vi "Gyro Example.vi"() -> ()   [LabVIEW 2011]
doc: "Gyro Example\n\nThis VI shows the user how to open a channel to a Gyro, get an angle from a gyro, and reinitialize the gyro."
uses:
  <vilib>/Rock Robotics/SystemInterfaces/AI/FPGA_AIGyroChannel.ctl
  <vilib>/Rock Robotics/WPI/Joystick/WPI_JoystickDeviceEnum.ctl
  <vilib>/Rock Robotics/WPI/RobotDrive/WPI_RobotDriveOpen4MotorWithCANJaguar.vi
  <vilib>/Rock Robotics/WPI/RobotDrive/WPI_RobotDriveArcadeDrive_Standard(NoSaturation).vi
panel:
  out "X-Axis Out":dbl(slide) scale=-1.0..1.0
  in  "Analog Channel":T1=enum."AI 2"
  in  "Gain (VoltsPerDegree/Second)":dbl=0.0068
  in  "stop":bool
  out "Angle":dbl(knob) scale=0.0..360.0
  in  "Reset Zero Position":bool
  # "This will display the current gyro angle."
  # "Wiring Diagram for Analog Breakout connected to an NI 9201"
  # "Set these inputs before running."
  # "This can be set while running."
  # "jumper to read battery or AI8"
  # "GND"
  # "SIG"
  # "5V"
  # "AI8\nAI7\nAI6\nAI5\nAI4\nAI3\nAI2\nAI1"
  # "Generic Gyro"
  # "+"
  # "12V from battery"
  # "-"
  # "default 0.0125\n0.00665 - close (within ~3 deg of 90 rot)\n0.00680 - (within ~19 of 360 rot)"
  # "\"power good\" LED"
  # "Specific Gyro Wiring:\nFor Analog Devices ADXRS401EB, ADXRS150EB and ADXRS300EB, wire RATEOUT to AI1 SIG (white PWM wire), wire AGND to AI1 GND (black PWM wire), and wire AVCC to AI1 5V (PWM red wire).  Also wire from AVCC to PDD.\n\nMost SparkFun Gyros wire according to the generic diagram"
  # "RATE"
  # "5V"
  # "GND"
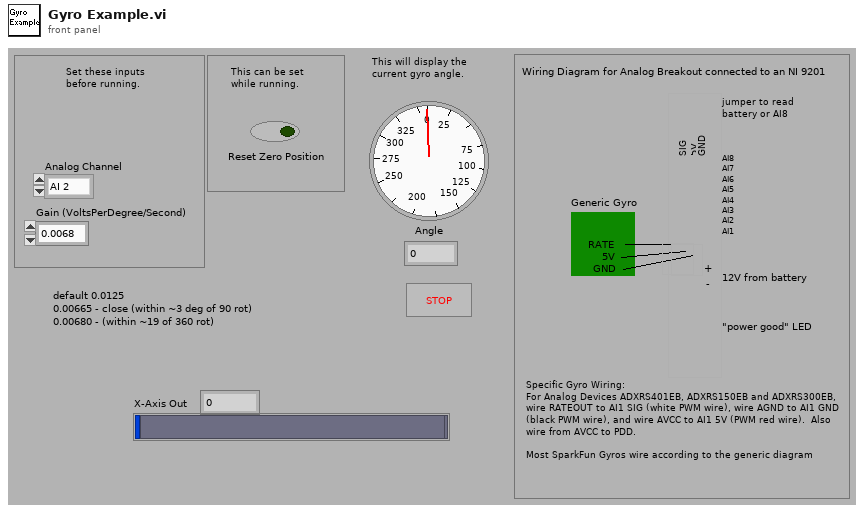
[diagram p1: front panel]
types:
  T1 = typedef "FPGA_AIGyroChannel.ctl" = enum8{"AI 1", "AI 2", "Invalid"}
  T2 = typedef "WPI_JoystickDeviceEnum.ctl" = enum16{"USB 1", "USB 2", "USB 3", "USB 4", "Kinect 1", "Kinect 2"}
  T3 = typedef "WPI_RobotDriveDevRef.ctl" = cluster{"DevStatus":errorcluster, "Motors[]":T4[], "Square Inputs":bool, "Max Output":dbl, "Isochronous":bool}
  T4 = typedef "WPI_MotorControlDeviceRef.ctl" = cluster{"DeviceStatus":errorcluster, "Type":enum16{"PWM", "CAN"}, "PWM":cluster{"Digital Module":T5, "PWM Channel":T6, "DeadBand":T7}, "CAN":cluster{"Device Number":u8, "Control Mode":T8, "Semaphore":T9, "Max Vout":dbl}, "Invert":bool, "TransformRef":T10, "InvTransformRef":T10}
  T5 = typedef "FPGA_TypedefDigitalModule.ctl" = enum16{"Digital Module 1", "Digital Module 2"}
  T6 = typedef "FPGA_DIOPWMChannel.ctl" = enum8{"PWM 1", "PWM 2", "PWM 3", "PWM 4", "PWM 5", "PWM 6", "PWM 7", "PWM 8", "PWM 9", "PWM 10", "Invalid"}
  T7 = typedef "WPI_PWMDeadband.ctl" = cluster{"Name":string, "maxPositivePwm":i32, "minPositivePwm":i32, "centerPwm":i32, "maxNegativePwm":i32, "minNegativePwm":i32, "angularRange":u16}
  T8 = typedef "WPI_CANJaguar_ControlMode.ctl" = enum8{"Percent VBus", "Current", "Speed", "Position", "Voltage"}
  T9 = typedef "Semaphore RefNum" = refnum<k1>
  T10 = typedef "WPI_PWMTransform_ConPane.ctl" = refnum<vi>
  T11 = typedef "WPI_GyroDevRef.ctl" = cluster{"DevStatus":errorcluster, "Analog Module":T12, "Analog Channel":T13, "Offset":dbl, "Gain (VoltsPerDegree/Second)":dbl}
  T12 = typedef "FPGA_TypedefAnalogModule.ctl" = enum16{"Analog Module 1", "Analog Module 2"}
  T13 = typedef "FPGA_AIChannel.ctl" = enum8{"AI 1", "AI 2", "AI 3", "AI 4", "AI 5", "AI 6", "AI 7", "AI 8", "Invalid"}
  T14 = typedef "WPI_JoystickDevRef.ctl" = cluster{"Device":T2}
  T15 = cluster{"axis 1 (x)":dbl, "axis 2 (y)":dbl, "axis 3 (throttle)":dbl, "axis 4":dbl, "axis 5":dbl, "axis 6":dbl}
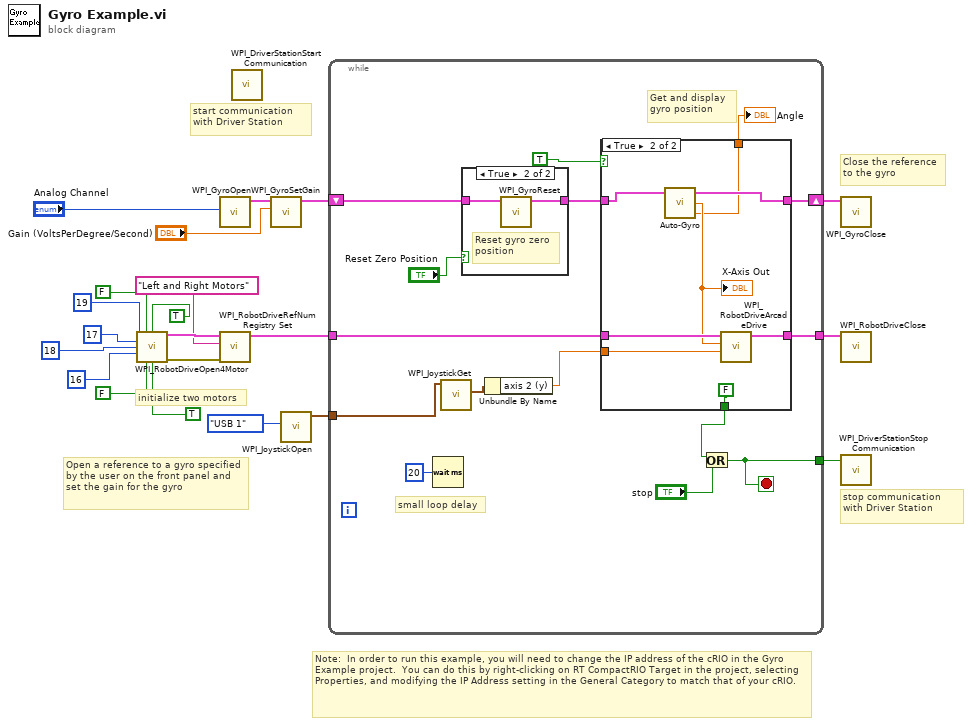
[diagram p0: block diagram]
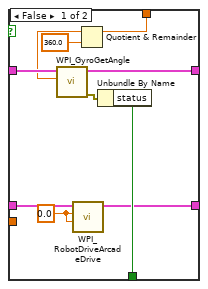
[diagram p2: hidden frame]
diagram:
  # "initialize two motors"
  # "stop communication with Driver Station"
  # "start communication with Driver Station"
  # "Note:  In order to run this example, you will need to change the IP address of the cRIO in the Gyro Example project.  You can do this by right-clicking on RT CompactRIO Target in the project, selecting Properties, and modifying the IP Address setting in the General Category to match that of your cRIO."
  # "Close the reference\nto the gyro"
  # "Open a reference to a gyro specified by the user on the front panel and set the gain for the gyro"
  n1 = call-poly <vilib>:"WPI_RobotDriveOpen4Motor.vi"("Rear Left Motor"=u8 19, "Rear Left Motor Inverted"=FALSE, "Rear Right Motor Inverted"=TRUE ("Rear Left Motor Inverted"), "Rear Right Motor"=u8 17, "Front Left Motor"=u8 18, "Front Right Motor"=u8 16, "Front Left Motor Inverted"=FALSE, "Front Right Motor Inverted"=TRUE) -> ("RobotDriveDevRef"=w15:T3, "error out"=w13:errorcluster)  [unwired: 6 in]
  n2 = call <vilib>:"WPI_GyroOpen.vi"("Analog Channel"="Analog Channel") -> ("GyroDevRef"=w19:T11)  [unwired: 5 in, 5 out]
  n3 = call <vilib>:"WPI_RobotDriveRefNum Registry Set.vi"("error in (no error)"=w13, "refnum name"="Left and Right Motors", "RobotDriveDevRef"=w15) -> ("RobotDriveDevRef"=w4:T3)  [unwired: 8 out]
  n4 = call <vilib>:"WPI_DriverStationStart Communication.vi"() -> ()  [unwired: 1 in, 11 out]
  n5 = call <vilib>:"WPI_GyroSetGain.vi"("Gain (VoltsPerDegree/Second)"="Gain (VoltsPerDegree/Second)", "GyroDevRef"=w19) -> ("GyroDevRef"=w18:T11)  [unwired: 1 in, 8 out]
  n6 = call <vilib>:"WPI_JoystickOpen.vi"("JoystickDevice"=WPI_JoystickDeviceEnum."USB 1") -> ("JoystickDevRef"=w1:T14)  [unwired: 10 in]
  n7 = while {
    shift-right: [w34] -> w21
    shift-left: w18 -> [w30]
    tunnel: [w33] -> w20
    tunnel: [w27] -> w3
    tunnel: w4 -> [w26]
    tunnel: w1 -> [w25]
    stop <- w33 stop-if-true
    # "small loop delay"
    # "Get and display\ngyro position"
    n8 = Wait (ms)(milliseconds to wait=u32 20) -> ()  [unwired: 1 out]
    n9 = call <vilib>:"WPI_JoystickGet.vi"("JoystickDevRef"=w25) -> ("Axes"=w24:T15)  [unwired: 4 in, 2 out]
    n10 = case shown="True" "Reset Zero Position" {
      tunnel: w30 -> [w55 w57]
      tunnel: [w55 w56] -> w35
      frame False {
      }
      frame True {
        # "Reset gyro zero \nposition"
        n11 = call <vilib>:"WPI_GyroReset.vi"("GyroDevRef"=w57) -> ("GyroDevRef"=w56:T11)  [unwired: 10 out]
      }
    }
    n12 = Unbundle By Name(w24) -> ("axis 2 (y)"=w23:dbl)
    n13 = case shown="True" TRUE ("Drive Straight") {
      tunnel: w35 -> [w46 w50]
      tunnel: [w44 w49] -> w34
      tunnel: [w42 w47] -> w29
      tunnel: [w40 FALSE ("status")] -> w28
      tunnel: [w38 w52] -> w27
      tunnel: w26 -> [w39 w53]
      tunnel: w23 -> [_ w51]
      frame False {
        w37 = 0.0 ("X axis value")
        n14 = call <vilib>:"WPI_GyroGetAngle.vi"("GyroDevRef"=w46) -> ("error out"=w41:errorcluster, "Angle"=w45:dbl, "GyroDevRef"=w44:T11)  [unwired: 1 in, 7 out]
        n15 = call-poly <vilib>:"WPI_RobotDriveArcadeDrive.vi"("Y axis value"=w37, "X axis value"=w37, "RobotDriveDevRef"=w39) -> ("RobotDriveDevRef"=w38:T3)  [unwired: 7 in, 1 out]
        n16 = Quotient & Remainder(x=w45, y=360.0) -> (x-y*floor(x/y)=w42:dbl)  [unwired: 1 out]
        n17 = Unbundle By Name(w41) -> ("status"=w40:bool)
      }
      frame True {
        n18 = call "Auto-Gyro.vi"("GyroDevRef"=w50) -> ("Angle"=w47:dbl, "X-Axis Out"=w48:dbl, "GyroDevRef Out"=w49:T11)  [unwired: 2 in]
        "X-Axis Out" <- w48
        n19 = call-poly <vilib>:"WPI_RobotDriveArcadeDrive.vi"("Y axis value"=w51, "X axis value"=w48, "RobotDriveDevRef"=w53) -> ("RobotDriveDevRef"=w52:T3)  [unwired: 7 in, 1 out]
      }
    }
    "Angle" <- w29
    n20 = Or(x=w28, y="stop") -> (x .or. y?=w33:bool)
  }
  n21 = call <vilib>:"WPI_GyroClose.vi"("GyroDevRef"=w21) -> ()  [unwired: 1 in, 10 out]
  n22 = call <vilib>:"WPI_RobotDriveClose.vi"("RobotDriveDevRef"=w3) -> ()  [unwired: 10 in, 1 out]
  n23 = call <vilib>:"WPI_DriverStationStop Communication.vi"("StopCommunication"=w20) -> ()  [unwired: 1 in, 10 out]
